vi "Draw Axes.vi"(8 "error in (no error)":errorcluster, 9 "Show Axes":bool, 10 "WFGraph Refnum":refnum<vi>, 11 "Display State In":T1={"Show Axes"=FALSE, "Show Y=0"=FALSE, "Controls"={"Type"=enum."Sine", "Periods"=0.0, "Points"=0, "Offset"=0.0, "Amplitdue"=0.0, "Starting Phase"=0.0, "func"=""}, "Show Current Location"=FALSE, "Current Location"=0, "dt"=0.0, "t0"=timestamp(0 s since 1904-01-01)} caption="State") -> (0 "error out":errorcluster, 3 "Display State Out":T1={"Show Axes"=FALSE, "Show Y=0"=FALSE, "Controls"={"Type"=enum."Sine", "Periods"=0.0, "Points"=0, "Offset"=0.0, "Amplitdue"=0.0, "Starting Phase"=0.0, "func"=""}, "Show Current Location"=FALSE, "Current Location"=0, "dt"=0.0, "t0"=timestamp(0 s since 1904-01-01)} caption="State")   [LabVIEW 2011, in "Waveform Control.xctl"]
uses:
  Waveform Control.xctl
  Controls/Waveform State.ctl
  FP Controls.ctl
  Function Types.ctl
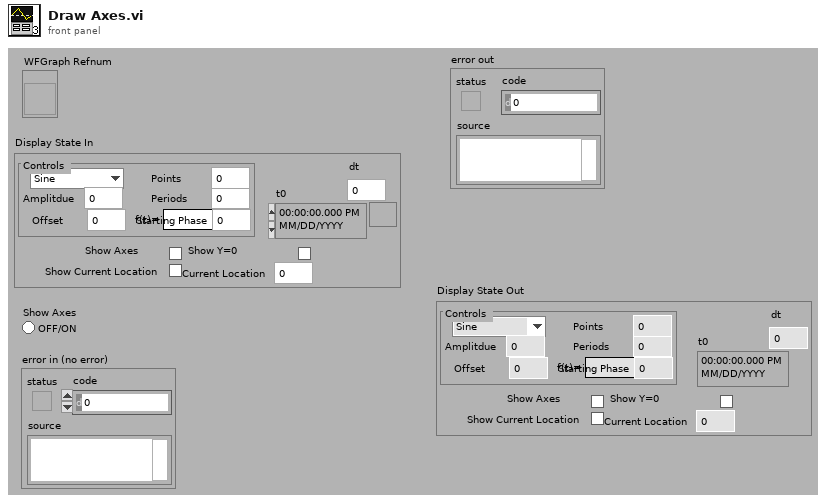
[diagram p1: front panel]
types:
  T1 = typedef "Waveform Control.xctl/Waveform State.ctl" = cluster{"Show Axes":bool, "Show Y=0":bool, "Controls":T2, "Show Current Location":bool, "Current Location":i32, "dt":dbl, "t0":timestamp}
  T2 = typedef "Waveform Control.xctl/FP Controls.ctl" = cluster{"Type":T3, "Periods":dbl, "Points":i32, "Offset":dbl, "Amplitdue":dbl, "Starting Phase":dbl, "func":string}
  T3 = typedef "Waveform Control.xctl/Function Types.ctl" = enum16{"Level", "Sine", "Triangle", "Ramp", "Saw Tooth", "Square", "Function"}
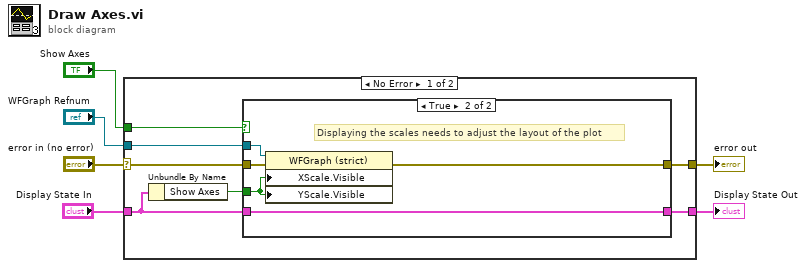
[diagram p0: block diagram]
diagram:
  n1 = case shown="No Error" "error in (no error)" {
    selector: "error in (no error)" -> [w13 w22]
    tunnel: [w12 w22] -> w5
    tunnel: "Show Axes" -> [w11 _]
    tunnel: "WFGraph Refnum" -> [w9 _]
    tunnel: [w8 w21] -> w2
    tunnel: "Display State In" -> [w7 w21]
    frame No Error {
      n2 = Unbundle By Name(w7) -> ("Show Axes"=w10:bool)
      n3 = case shown="True" w11 {
        tunnel: w10 -> [_ w20]
        tunnel: [w14 w19] -> w12
        tunnel: w13 -> [w14 w18]
        tunnel: w9 -> [_ w17]
        tunnel: [w15 w16] -> w8
        tunnel: w7 -> [w15 w16]
        frame False {
        }
        frame True {
          # "Displaying the scales needs to adjust the layout of the plot"
          n4 = property on="Property Node" class="WFGraph (strict)"(reference=w17, error in=w18, "XScale.Visible"=w20, "YScale.Visible"=w20) -> (error out=w19:errorcluster)  [unwired: 1 out]
        }
      }
    }
    frame Error {
    }
  }
  "error out" <- w5
  "Display State Out" <- w2
